vi "Read.vi"(8 "error in (no error)":errorcluster, 10 "Symbol Name":string, 11 "TwinCAT ADS in":refnum<class "TwinCAT ADS.lvclass">) -> (0 "error out":errorcluster, 1 "Value":variant, 3 "TwinCAT ADS out":refnum<class "TwinCAT ADS.lvclass">)   [LabVIEW 2018, in "TwinCAT ADS.lvclass"]
uses:
  TwinCAT ADS.lvclass
  TwinCAT ADS.lvclass/TwinCAT ADS.ctl
  TwinCAT.Ads
  Get From Symbol Map.vi
  Get From Symbol Map Daemon.vi
  Get Symbol Map.vi
  Format String.vi
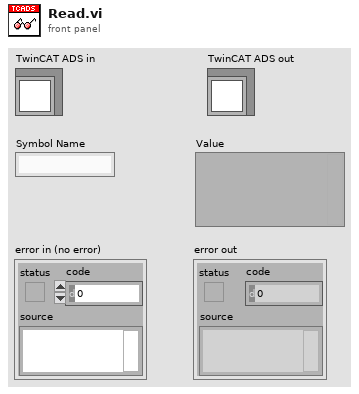
[diagram p1: front panel]
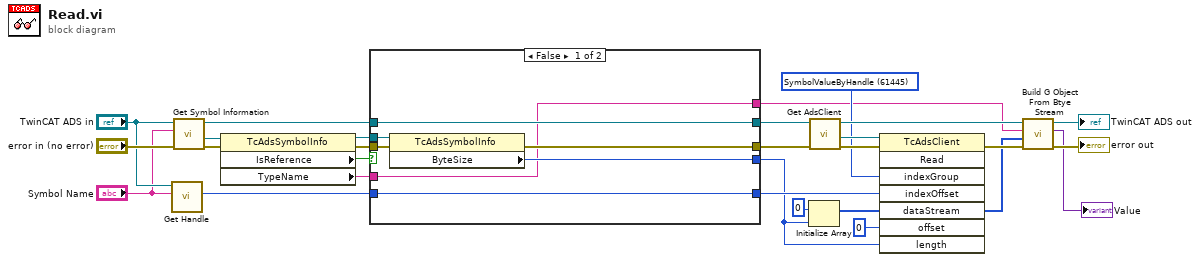
[diagram p0: block diagram]
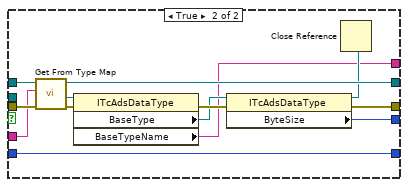
[diagram p2: hidden frame]
diagram:
  w19 = u32 61445 items=["PlcRWIB"=16384, "PlcRWOB"=16400, "PlcRWMB"=16416, "PlcRWRB"=16432, "PlcRWDB"=16448, "SymbolTable"=61440, "SymbolName"=61441, "SymbolValue"=61442, "SymbolHandleByName"=61443, "SymbolValueByName"=61444, "SymbolValueByHandle"=61445, "SymbolReleaseHandle"=61446, "SymbolInfoByName"=61447, "SymbolVersion"=61448, "SymbolInfoByNameEx"=61449, "SymbolDownload"=61450, "SymbolUpload"=61451, "SymbolUploadInfo"=61452, "SymbolNote"=61456, "IOImageRWIB"=61472, "IOImageRWIX"=61473, "IOImageRWOB"=61488, "IOImageRWOX"=61489, "IOImageClearI"=61504, "IOImageClearO"=61520, "SumCommandRead"=61568, "SumCommandWrite"=61569, "SumCommandReadWrite"=61570, "SumCommandReadEx"=61571, "SumCommandReadEx2"=61572, "SumCommandAddDevNote"=61573, "SumCommandDelDevNote"=61574, "DeviceData"=61696] ("SumCommandRead")
  n1 = call "Get Handle.vi"("Symbol Name"="Symbol Name", "TwinCAT ADS in"="TwinCAT ADS in") -> ("Handle"=w4:i32)  [unwired: 7 in, 2 out]
  n2 = call "Get Symbol Information.vi"("error in (no error)"="error in (no error)", "Symbol Name"="Symbol Name", "TwinCAT ADS in"="TwinCAT ADS in") -> ("error out"=w9:errorcluster, ".NET Symbol Information"=w8:refnum<k24>, "TwinCAT ADS out"=w7:refnum<class "TwinCAT ADS.lvclass">)  [unwired: 6 in]
  n3 = property class="TcAdsSymbolInfo"(reference=w8, error in=w9) -> (reference out=w10:refnum<k24>, error out=w12:errorcluster, "IsReference"=w13:bool, "TypeName"=w11:string)
  n4 = case shown="False" w13 {
    tunnel: w12 -> [w35 w48]
    tunnel: [w31 w44] -> w6
    tunnel: w11 -> [w30 w45]
    tunnel: [w30 w37] -> w2
    tunnel: [w32 w41] -> w1
    tunnel: [w33 w39] -> w5
    tunnel: w10 -> [w34 _]
    tunnel: w7 -> [w31 w38]
    tunnel: w4 -> [w29 w36]
    tunnel: [w29 w36] -> w3
    frame False {
      n5 = property class="TcAdsSymbolInfo"(reference=w34, error in=w35) -> (error out=w33:errorcluster, "ByteSize"=w32:i32)  [unwired: 1 out]
    }
    frame True {
      n6 = call "Get From Type Map.vi"("error in (no error)"=w48, "Type Name"=w45, "TwinCAT ADS in"=w38) -> ("error out"=w47:errorcluster, ".NET AdsDataType"=w46:refnum<k24>, "TwinCAT ADS out"=w44:refnum<class "TwinCAT ADS.lvclass">)  [unwired: 6 in]
      n7 = property class="ITcAdsDataType"(reference=w46, error in=w47) -> (error out=w43:errorcluster, "BaseType"=w42:refnum<k24>, "BaseTypeName"=w37:string)  [unwired: 1 out]
      n8 = property class="ITcAdsDataType"(reference=w42, error in=w43) -> (reference out=w40:refnum<k24>, error out=w39:errorcluster, "ByteSize"=w41:i32)
      n9 = Close Reference(reference=w40) -> ()  [unwired: 1 in, 1 out]
    }
  }
  n10 = Initialize Array(u8 0, w1) -> (w23:u8[])
  n11 = call "Get AdsClient.vi"("error in (no error)"=w5, "TwinCAT ADS in"=w6) -> ("error out"=w27:errorcluster, ".NET TcAdsClient"=w26:refnum<k24>, "TwinCAT ADS out"=w25:refnum<class "TwinCAT ADS.lvclass">)  [unwired: 7 in]
  n12 = invoke class="TcAdsClient" method="Read"(reference=w26, error in=w27, "indexGroup"=w19, "indexOffset"=w3, "dataStream"=w23, "offset"=0, "length"=w1) -> (error out=w21:errorcluster, "dataStream"=w20:u8[])  [unwired: 1 in, 6 out]
  n13 = call "Build G Object From Btye Stream.vi"("error in (no error)"=w21, "Byte Stream in"=w20, "Type Name"=w2, "TwinCAT ADS in"=w25) -> ("error out"=→"error out":errorcluster, "Value"=→"Value":variant, "TwinCAT ADS out"=→"TwinCAT ADS out":refnum<class "TwinCAT ADS.lvclass">)  [unwired: 4 in, 1 out]
